vi "Jumpstart.vi"() -> ()   [LabVIEW 2019]
uses:
  <vilib>/Analysis/NI_AALPro.lvlib
panel:
  out "subarray":dbl[][](array[numeric])
  in  "Array":dbl[][](array[numeric])
  out "!A":bool
  out "A || B":bool
  out "A && B":bool
  out "String 2":string
  in  "Combo Box":string(combo)
  in  "String":string
  in  "C_bool":bool
  in  "B_bool":bool
  in  "A_bool":bool
  in  "C":dbl(knob) scale=0.0..10.0
  in  "B":dbl(slide) scale=0.0..10.0
  in  "A":dbl
  # "Numeric Inputs"
  # "Boolean Inputs"
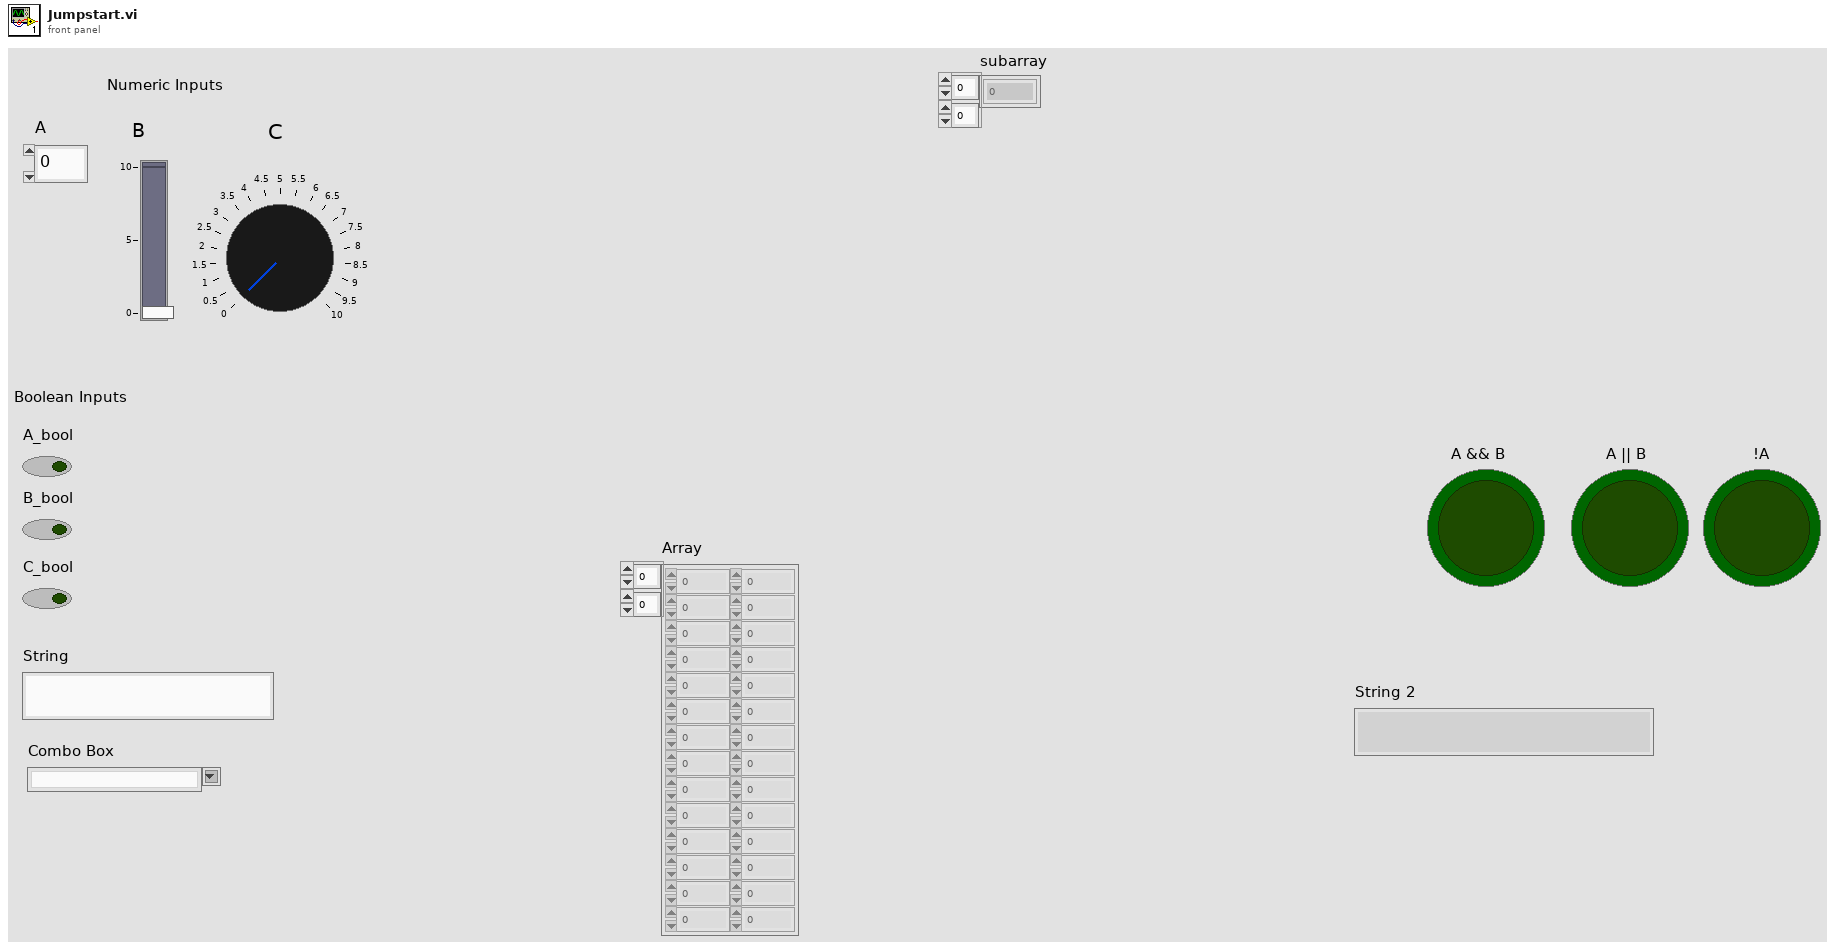
[diagram p1: front panel]
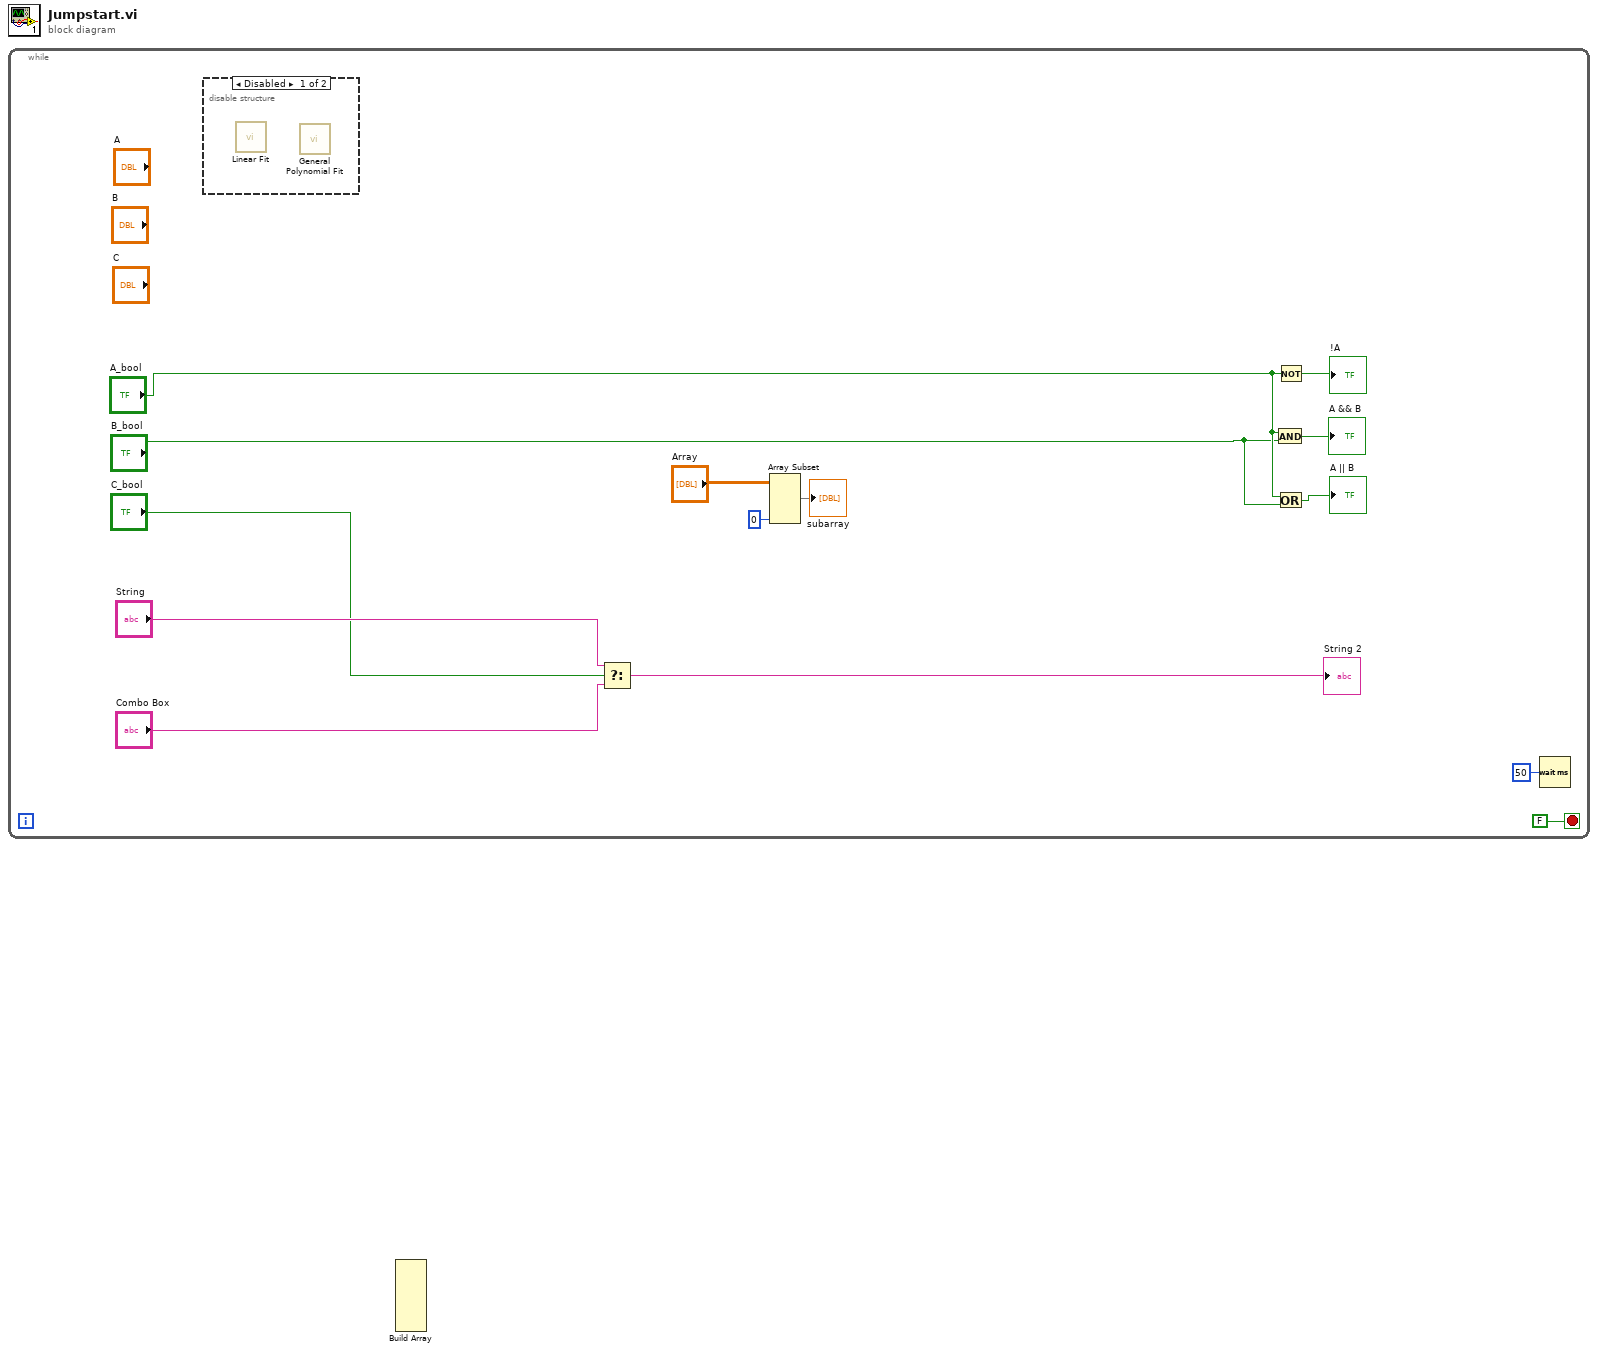
[diagram p0: block diagram]
diagram:
  n1 = while {
    stop <- FALSE stop-if-true
    n2 = disable-structure shown="Disabled" {
      frame Disabled {
        n3 = call <vilib>:"Linear Fit.vi"() -> ()  [unwired: 11 in, 5 out]
        n4 = call <vilib>:"General Polynomial Fit.vi"() -> ()  [unwired: 12 in, 4 out]
      }
      frame Enabled {
      }
    }
    n5 = Select(t="String", s="C_bool", f="Combo Box") -> (s? t:f=→"String 2":string)
    n6 = Array Subset(array="Array", length (col)=0 ("length")) -> (→"subarray":dbl[][])  [unwired: 3 in]
    n7 = And(x="A_bool", y="B_bool") -> (x .and. y?=→"A && B":bool)
    n8 = Not(x="A_bool") -> (.not. x?=→"!A":bool)
    n9 = Or(x="A_bool", y="B_bool") -> (x .or. y?=→"A || B":bool)
    n10 = Wait (ms)(milliseconds to wait=u32 50) -> ()  [unwired: 1 out]
  }
  n11 = Build Array() -> ()  [unwired: 9 in, 1 out]
